vi "Write Table_Ref.vi"(8 "error in (no error)":errorcluster, 10 "Table_Ref":refnum<vi>, 11 "Multimeter in":refnum<class "Multimeter.lvclass">) -> (0 "error out":errorcluster, 3 "Multimeter out":refnum<class "Multimeter.lvclass">)   [LabVIEW 2019, in "Multimeter.lvlib" / "Multimeter.lvclass"]
uses:
  Library/Multimeter.lvclass
  Library/Multimeter.lvclass/Multimeter.ctl
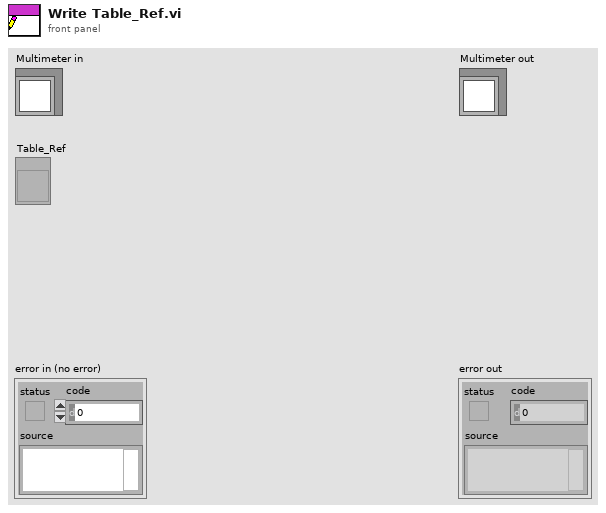
[diagram p1: front panel]
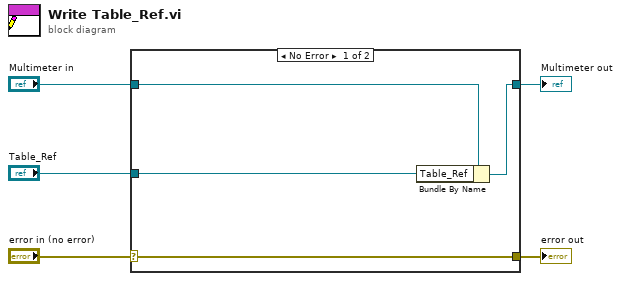
[diagram p0: block diagram]
diagram:
  n1 = case shown="No Error" "error in (no error)" {
    selector: "error in (no error)" -> [w9 w10]
    tunnel: [w9 w10] -> w4
    tunnel: [w7 w11] -> w2
    tunnel: "Multimeter in" -> [w8 w11]
    tunnel: "Table_Ref" -> [w6 _]
    frame No Error {
      n2 = Bundle By Name(cluster=w8, "Table_Ref"=w6) -> (w7:refnum<class "Multimeter.lvclass">)
    }
    frame Error {
    }
  }
  "error out" <- w4
  "Multimeter out" <- w2
